vi "Simple Dataflow Example.vi"() -> ()   [LabVIEW 2013]
uses:
  lightfield-automation-labview/LightField Automation.lvclass
panel:
  in  "ExperimentName":string
  in  "Acquire":bool
  out "Acquire ROI 1, Frame 1, Row 1":dbl[](graph)
  out "Capture ROI 1, Frame 1, Row 1":dbl[](graph)
  in  "Capture":bool
  out "Acquire ROI 1, Frame 1":dbl[][](graph)
  out "Capture ROI 1, Frame 1":dbl[][](graph)
  in  "?":bool
  out "Exposures Per Frame":i32
  in  "Exposures Per Frame":i32=1
  out "Number of Frames":i32
  in  "Number of Frames":i32=1
  out "Exposure Time (s)":dbl
  in  "Exposure Time (s)":dbl=0.1
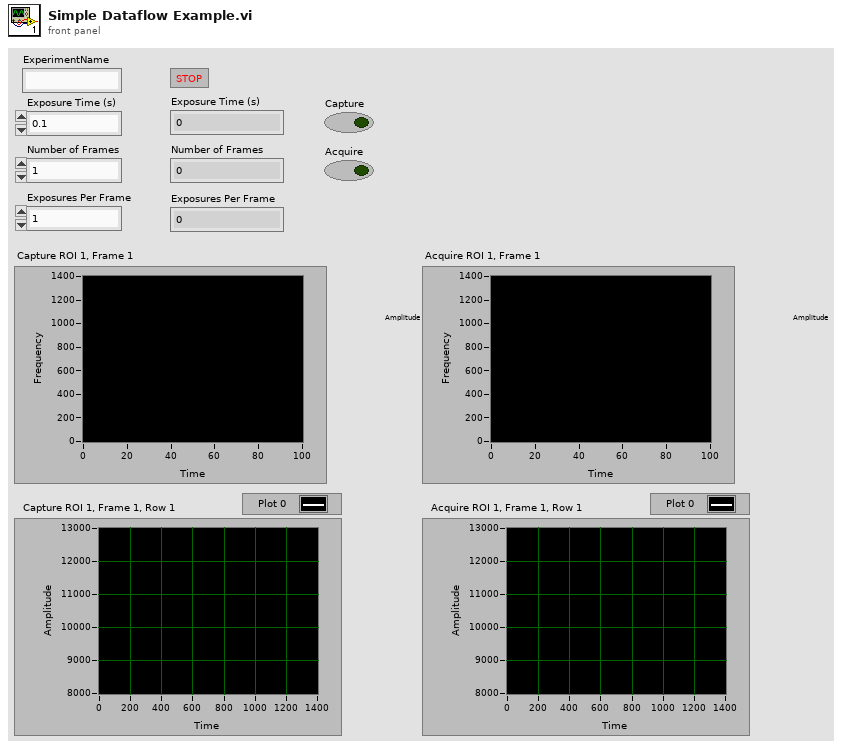
[diagram p1: front panel]
types:
  T1 = cluster{"Image":dbl[][][], "Frame Size":cluster{"F":i32, "Y":i32, "X":i32}}[]
  T2 = cluster{"Image":dbl[][][], "Frame Size":cluster{"F":i32, "Y":i32, "X":i32}}
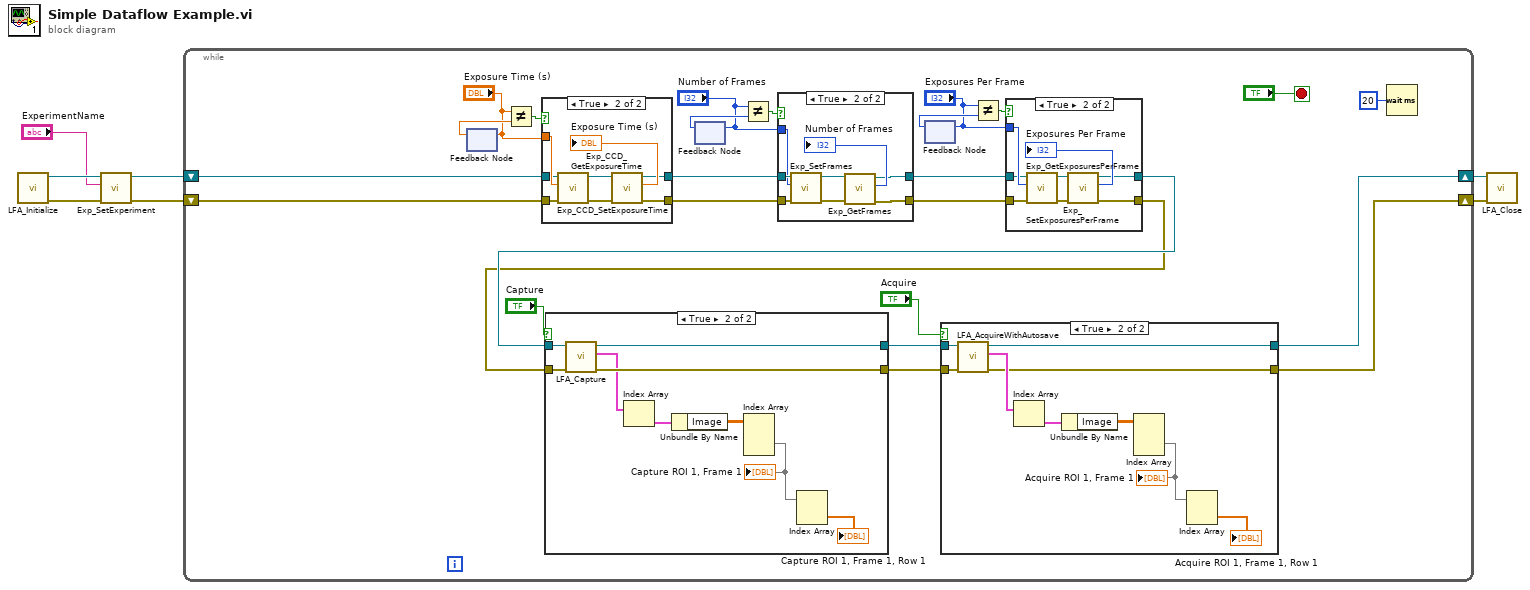
[diagram p0: block diagram]
diagram:
  n1 = call "LFA_Initialize.vi"() -> ("error out"=w6:errorcluster, "LightField Automation out"=w7:refnum<class "LightField Automation.lvclass">)  [unwired: 10 in]
  n2 = call "Exp_SetExperiment.vi"("error in (no error)"=w6, "ExperimentName"="ExperimentName", "LightField Automation in"=w7) -> ("error out"=w4:errorcluster, "LightField Automation out"=w3:refnum<class "LightField Automation.lvclass">)  [unwired: 7 in]
  n3 = while {
    shift-right: [w12] -> w1
    shift-left: w3 -> [w8]
    shift-right: [w11] -> w2
    shift-left: w4 -> [w9]
    stop <- "?" stop-if-true
    n4 = feedback-in #1("Exposure Time (s)") -> ()
    n5 = feedback #1() -> (w29:dbl)  [unwired: 1 in]
    n6 = Not Equal?(x="Exposure Time (s)", y=w29) -> (x != y?=w30:bool)
    n7 = case shown="True" w30 {
      tunnel: "Exposure Time (s)" -> [_ w81]
      tunnel: w8 -> [w75 w80]
      tunnel: w9 -> [w76 w79]
      tunnel: [w75 w78] -> w27
      tunnel: [w76 w77] -> w26
      frame False {
      }
      frame True {
        n8 = call "Exp_CCD_SetExposureTime.vi"("error in (no error)"=w79, "Exposure Time (s)"=w81, "LightField Automation in"=w80) -> ("error out"=w82:errorcluster, "LightField Automation out"=w83:refnum<class "LightField Automation.lvclass">)  [unwired: 7 in]
        n9 = call "Exp_CCD_GetExposureTime.vi"("error in (no error)"=w82, "LightField Automation in"=w83) -> ("error out"=w77:errorcluster, "Exposure Time (s)"=→"Exposure Time (s)":dbl, "LightField Automation out"=w78:refnum<class "LightField Automation.lvclass">)  [unwired: 7 in]
      }
    }
    n10 = feedback #2() -> (w25:i32)  [unwired: 1 in]
    n11 = feedback-in #2("Number of Frames") -> ()
    n12 = Not Equal?(x="Number of Frames", y=w25) -> (x != y?=w24:bool)
    n13 = case shown="True" w24 {
      tunnel: w27 -> [w66 w71]
      tunnel: w26 -> [w65 w70]
      tunnel: "Number of Frames" -> [_ w69]
      tunnel: [w66 w68] -> w19
      tunnel: [w65 w67] -> w18
      frame False {
      }
      frame True {
        n14 = call "Exp_SetFrames.vi"("error in (no error)"=w70, "Number of Frames"=w69, "LightField Automation in"=w71) -> ("error out"=w73:errorcluster, "LightField Automation out"=w74:refnum<class "LightField Automation.lvclass">)  [unwired: 7 in]
        n15 = call "Exp_GetFrames.vi"("error in (no error)"=w73, "LightField Automation in"=w74) -> ("error out"=w67:errorcluster, "Frames"=→"Number of Frames":i32, "LightField Automation out"=w68:refnum<class "LightField Automation.lvclass">)  [unwired: 7 in]
      }
    }
    n16 = feedback #3() -> (w22:i32)  [unwired: 1 in]
    n17 = feedback-in #3("Exposures Per Frame") -> ()
    n18 = Not Equal?(x="Exposures Per Frame", y=w22) -> (x != y?=w21:bool)
    n19 = case shown="True" w21 {
      tunnel: "Exposures Per Frame" -> [_ w61]
      tunnel: w19 -> [w56 w60]
      tunnel: w18 -> [w55 w59]
      tunnel: [w55 w58] -> w15
      tunnel: [w56 w57] -> w17
      frame False {
      }
      frame True {
        n20 = call "Exp_SetExposuresPerFrame.vi"("error in (no error)"=w59, "Exposures Per Frame"=w61, "LightField Automation in"=w60) -> ("error out"=w64:errorcluster, "LightField Automation out"=w63:refnum<class "LightField Automation.lvclass">)  [unwired: 7 in]
        n21 = call "Exp_GetExposuresPerFrame.vi"("error in (no error)"=w64, "LightField Automation in"=w63) -> ("error out"=w58:errorcluster, "Exposures Per Frame"=→"Exposures Per Frame":i32, "LightField Automation out"=w57:refnum<class "LightField Automation.lvclass">)  [unwired: 7 in]
      }
    }
    n22 = case shown="True" "Capture" {
      tunnel: w17 -> [w45 w47]
      tunnel: w15 -> [w44 w46]
      tunnel: [w45 w49] -> w14
      tunnel: [w44 w50] -> w13
      frame False {
      }
      frame True {
        n23 = call "LFA_Capture.vi"("error in (no error)"=w46, "LightField Automation in"=w47) -> ("error out"=w50:errorcluster, "Data"=w48:T1, "LightField Automation out"=w49:refnum<class "LightField Automation.lvclass">)  [unwired: 7 in]
        n24 = Index Array(array=w48) -> (element=w54:T2)  [unwired: 1 in]
        n25 = Unbundle By Name(w54) -> ("Image"=w53:dbl[][][])
        n26 = Index Array(array=w53) -> (element=w52:dbl[][])  [unwired: 3 in]
        "Capture ROI 1, Frame 1" <- w52
        n27 = Index Array(array=w52) -> (element=→"Capture ROI 1, Frame 1, Row 1":dbl[])  [unwired: 2 in]
      }
    }
    n28 = case shown="True" "Acquire" {
      tunnel: w14 -> [w34 w38]
      tunnel: w13 -> [w33 w39]
      tunnel: [w34 w37] -> w12
      tunnel: [w33 w35] -> w11
      frame False {
      }
      frame True {
        n29 = call "LFA_AcquireWithAutosave.vi"("error in (no error)"=w39, "LightField Automation in"=w38) -> ("error out"=w35:errorcluster, "Data"=w36:T1, "LightField Automation out"=w37:refnum<class "LightField Automation.lvclass">)  [unwired: 7 in]
        n30 = Index Array(array=w36) -> (element=w43:T2)  [unwired: 1 in]
        n31 = Unbundle By Name(w43) -> ("Image"=w42:dbl[][][])
        n32 = Index Array(array=w42) -> (element=w40:dbl[][])  [unwired: 3 in]
        "Acquire ROI 1, Frame 1" <- w40
        n33 = Index Array(array=w40) -> (element=→"Acquire ROI 1, Frame 1, Row 1":dbl[])  [unwired: 2 in]
      }
    }
    n34 = Wait (ms)(milliseconds to wait=u32 20) -> ()  [unwired: 1 out]
  }
  n35 = call "LFA_Close.vi"("error in (no error)"=w2, "LightField Automation in"=w1) -> ()  [unwired: 8 in, 2 out]
